vi "tearDown.vi"(8 "error in (no error)":errorcluster, 11 "reference in":refnum<class "Instrument Addon Scripting API Channels Unit Tests.lvclass">) -> (0 "error out":errorcluster, 3 "reference out":refnum<class "Instrument Addon Scripting API Channels Unit Tests.lvclass">)   [LabVIEW 2019, in "Instrument Addon Scripting API Channels Unit Tests.lvclass"]
doc: "tearDown runs after the test method has completed. Use this method to clean up any operations or references that were opened by setUp or the test method. Unit tests should be independent of other unit tests so this VI should ensure that the next test can run in a 'clean' test environment."
uses:
  Instrument Addon Scripting API Channels Unit Tests.lvclass
  Instrument Addon Scripting API Channels Unit Tests.lvclass/Instrument Addon Scripting API Channels Unit Tests.ctl
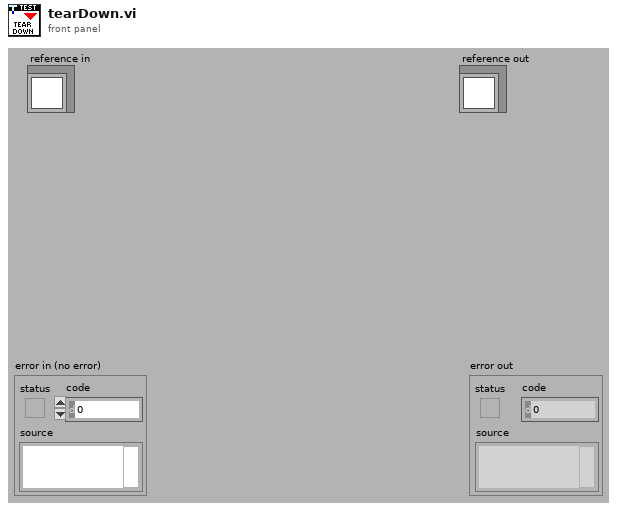
[diagram p1: front panel]
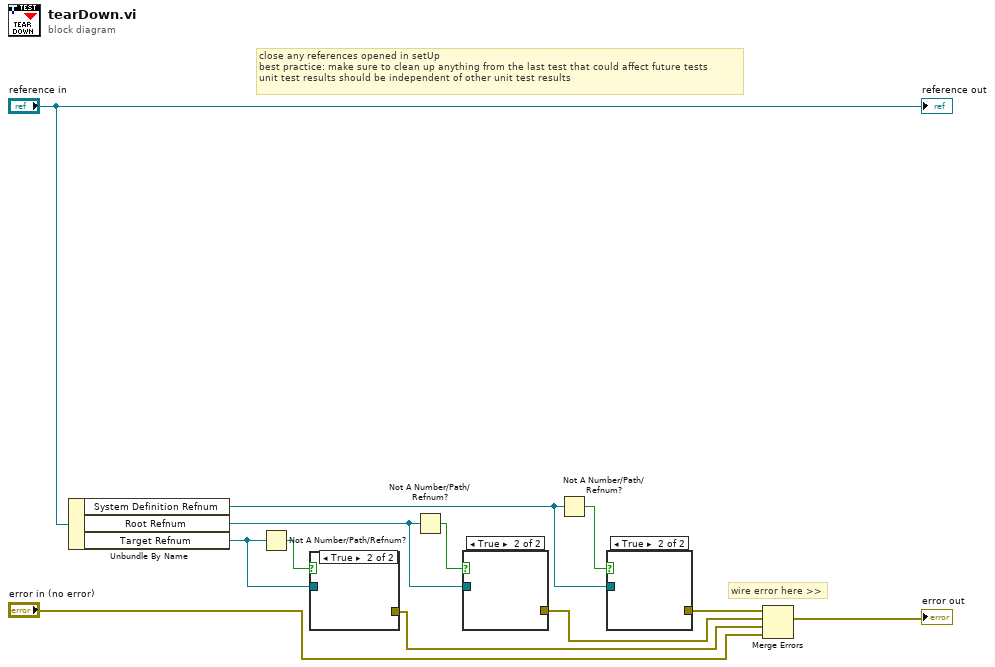
[diagram p0: block diagram]
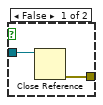
[diagram p2: hidden frame]
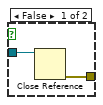
[diagram p3: hidden frame]
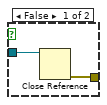
[diagram p4: hidden frame]
diagram:
  # "wire error here >>"
  # "close any references opened in setUp\nbest practice: make sure to clean up anything from the last test that could affect future tests\nunit test results should be independent of other unit test results"
  n1 = Unbundle By Name("reference in") -> ("System Definition Refnum"=w5:refnum<k24>, "Root Refnum"=w7:refnum<k24>, "Target Refnum"=w9:refnum<k24>)
  n2 = Not A Number/Path/Refnum?(number/path/refnum=w9) -> (NaN/Path/Refnum?=w10:bool)
  n3 = case shown="True" w10 {
    tunnel: w9 -> [w14 _]
    tunnel: [w13 _] -> w2
    frame False {
      n4 = Close Reference(reference=w14) -> (error out=w13:errorcluster)  [unwired: 1 in]
    }
    frame True {
    }
  }
  n5 = Not A Number/Path/Refnum?(number/path/refnum=w7) -> (NaN/Path/Refnum?=w8:bool)
  n6 = case shown="True" w8 {
    tunnel: w7 -> [w16 _]
    tunnel: [w15 _] -> w3
    frame False {
      n7 = Close Reference(reference=w16) -> (error out=w15:errorcluster)  [unwired: 1 in]
    }
    frame True {
    }
  }
  n8 = Not A Number/Path/Refnum?(number/path/refnum=w5) -> (NaN/Path/Refnum?=w6:bool)
  n9 = case shown="True" w6 {
    tunnel: w5 -> [w18 _]
    tunnel: [w17 _] -> w4
    frame False {
      n10 = Close Reference(reference=w18) -> (error out=w17:errorcluster)  [unwired: 1 in]
    }
    frame True {
    }
  }
  n11 = Merge Errors(w4, w3, w2, "error in (no error)") -> (→"error out":errorcluster)
  "reference out" <- "reference in"
